vi "SpinnySingleCameraTrigger.vi"(8 "error in":errorcluster, 9 "Stepper #":u8=1, 11 "Arduino Resource":T1={"VISA resource"="", "Board Type"=enum."Uno", "Connection Type"=enum."USB / Serial", "Bytes Per Packet (15)"=15}) -> (0 "error out":errorcluster, 3 "Arduino Resource Out":T1={"VISA resource"="", "Board Type"=enum."Uno", "Connection Type"=enum."USB / Serial", "Bytes Per Packet (15)"=15})   [LabVIEW 2014]
doc: "set the interval (in steps of the indicated stepper) for a pulse to be sent to the indicated pin."
uses:
  <vilib>/LabVIEW Interface for Arduino/Type Defs/Arduino Resource.ctl
  <vilib>/LabVIEW Interface for Arduino/Type Defs/Board Type.ctl
  <vilib>/LabVIEW Interface for Arduino/LabVIEW Interface for Arduino.lvlib
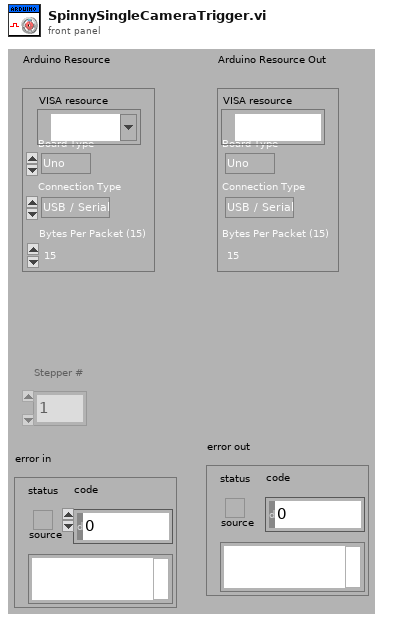
[diagram p1: front panel]
types:
  T1 = typedef "LabVIEW Interface for Arduino.lvlib/Arduino Resource.ctl" = cluster{"VISA resource":refnum<visa-resource-name>, "Board Type":T2, "Connection Type":enum8{"USB / Serial"}, "Bytes Per Packet (15)":u8}
  T2 = typedef "LabVIEW Interface for Arduino.lvlib/Board Type.ctl" = enum16{"Uno", "Dimuelanove w/Atmega 328", "Mega 2560"}
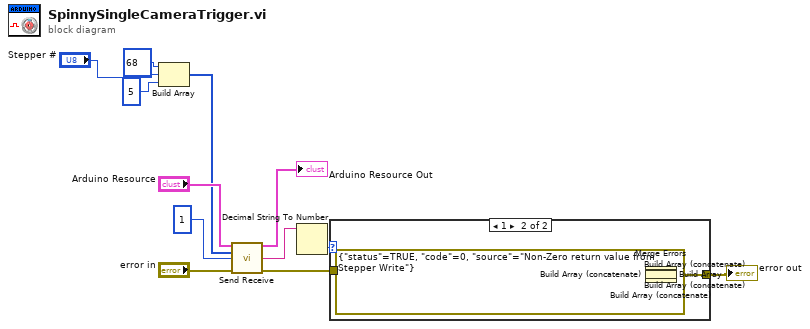
[diagram p0: block diagram]
diagram:
  n1 = Build Array(u8 68, "Stepper #", u8 5 ("element")) -> (w9:u8[])
  n2 = call <vilib>:"Send Receive.vi"("Arduino Resource"="Arduino Resource", "Data"=w9, "Bytes To Read (0)"=u8 1, "error in"="error in") -> ("Arduino Resource"=→"Arduino Resource Out":T1, "Read Buffer"=w3:string, "error out"=w4:errorcluster)  [unwired: 9 in]
  n3 = Decimal String To Number(string=w3) -> (number=w6:i32)  [unwired: 2 in, 1 out]
  n4 = case shown="1" w6 {
    tunnel: w4 -> [w13 w21]
    tunnel: [w13 w20] -> w5
    frame 0, Default {
    }
    frame 1 {
      n5 = Build Array(w21, errorcluster {"status"=TRUE, "code"=0, "source"="Non-Zero return value from Stepper Write"} ("error in")) -> (w18:errorcluster[])
      n6 = Build Array (concatenate)(w18) -> (w17:errorcluster[])
      n7 = Build Array (concatenate)(w17) -> (w16:errorcluster[])
      n8 = Build Array (concatenate)(w16) -> (w15:errorcluster[])
      n9 = Build Array (concatenate)(w15) -> (w14:errorcluster[])
      n10 = Merge Errors(w14) -> (w20:errorcluster)
    }
  }
  "error out" <- w5
